vi "data_grid_v128_create_basemap.vi"(8 "Y_spacing":dbl format="%#_13g", 9 "X_spacing":dbl format="%#_13g", 10 "No. Rows":i32=16, 11 "No. Columns":i32=8) -> (2 "Grids_Unbounded":cluster{dbl[][], dbl[][], dbl[][]}, 3 "Grids_Bounded":cluster{dbl[][], dbl[][], dbl[][]})   [LabVIEW 2018]
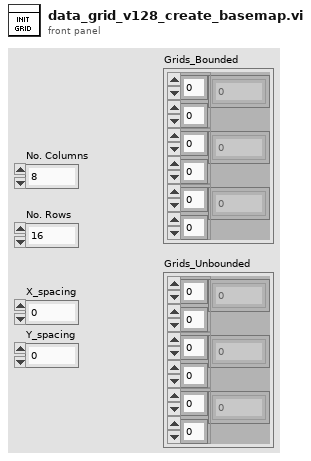
[diagram p1: front panel]
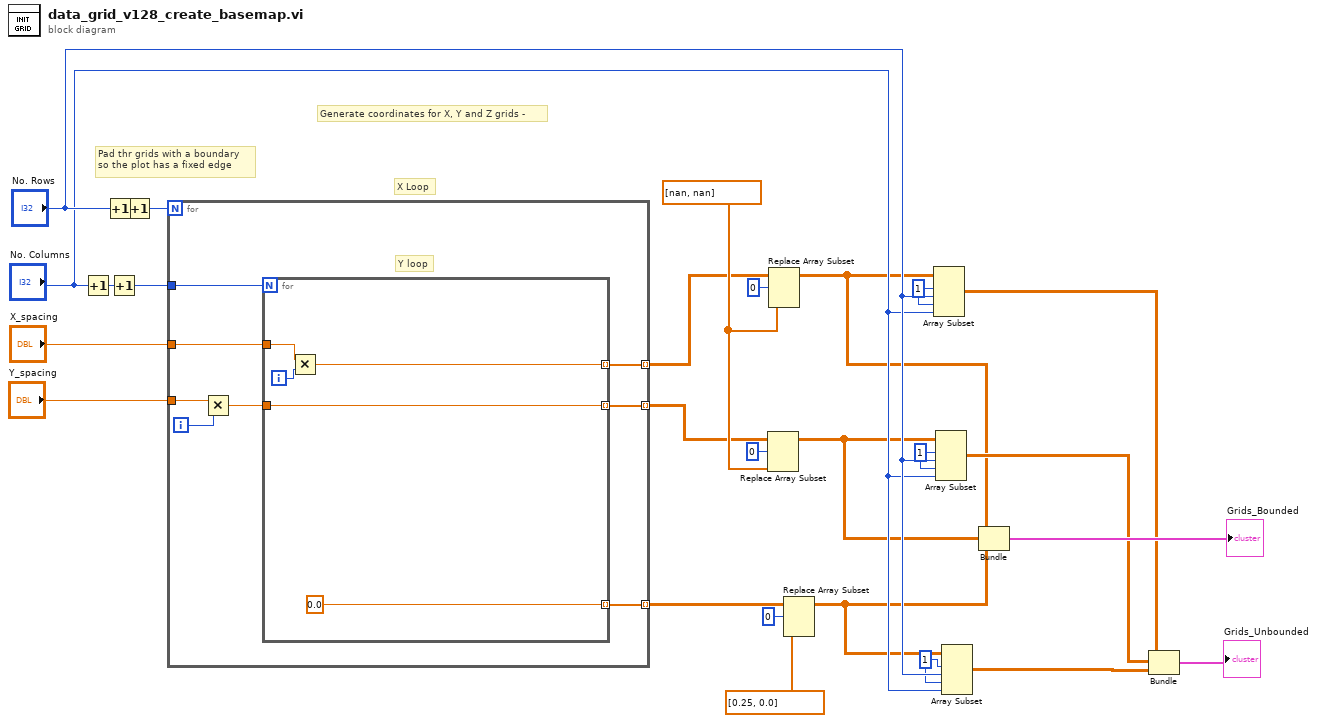
[diagram p0: block diagram]
diagram:
  w13 = dbl[] [nan, nan]
  w16 = 1 ("index")
  w19 = 1 ("index")
  w20 = 1 ("index")
  # "Pad thr grids with a boundary\nso the plot has a fixed edge"
  # "Generate coordinates for X, Y and Z grids -"
  # "X Loop"
  n1 = Increment(x="No. Columns") -> (x+1=w25:i32)
  n2 = Increment(x="No. Rows") -> (x+1=w27:i32)
  n3 = Increment(x=w25) -> (x+1=w24:i32)
  n4 = Increment(x=w27) -> (x+1=w26:i32)
  n5 = for {
    N: w26 -> [_]
    tunnel: [w35] -> w8 mode=indexing
    tunnel: w24 -> [w34]
    tunnel: "X_spacing" -> [w33]
    tunnel: "Y_spacing" -> [w31]
    tunnel: [w29] -> w4 mode=indexing
    tunnel: [w28] -> w2 mode=indexing
    i -> [w32]
    # "Y loop"
    n6 = Multiply(x=w31, y=w32) -> (x*y=w30:dbl)
    n7 = for {
      N: w34 -> [_]
      tunnel: [0.0 ("element")] -> w35 mode=indexing
      tunnel: w33 -> [w39]
      tunnel: w30 -> [w36]
      tunnel: [w37] -> w29 mode=indexing
      tunnel: [w36] -> w28 mode=indexing
      i -> [w38]
      n8 = Multiply(x=w39, y=w38) -> (x*y=w37:dbl)
    }
  }
  n9 = Replace Array Subset(array=w2, new element=w13, index (row)=0) -> (w1:dbl[][])  [unwired: 1 in]
  n10 = Replace Array Subset(array=w4, new element=w13, index (row)=0) -> (w3:dbl[][])  [unwired: 1 in]
  n11 = Replace Array Subset(array=w8, new element=dbl[] [0.25, 0.0], index (row)=0) -> (w7:dbl[][])  [unwired: 1 in]
  n12 = Array Subset(array=w3, index (row)=w20, length (row)="No. Rows", index (col)=w20, length (col)="No. Columns") -> (w5:dbl[][])
  n13 = Array Subset(array=w1, index (row)=w19, length (row)="No. Rows", index (col)=w19, length (col)="No. Columns") -> (w6:dbl[][])
  n14 = Array Subset(array=w7, index (row)=w16, length (row)="No. Rows", index (col)=w16, length (col)="No. Columns") -> (w9:dbl[][])
  n15 = Bundle(w3, w1, w7) -> (→"Grids_Bounded":cluster{dbl[][], dbl[][], dbl[][]})  [unwired: 1 in]
  n16 = Bundle(w5, w6, w9) -> (→"Grids_Unbounded":cluster{dbl[][], dbl[][], dbl[][]})  [unwired: 1 in]
